vi "Rotate Pattern.vi"(9 "Target":i32, 10 "Current":i32, 11 "Pattern In":bool[][](array[boolean])) -> (2 "Rotation CCW":i32, 3 "Pattern Out":bool[][](array[boolean]))   [LabVIEW 2020]
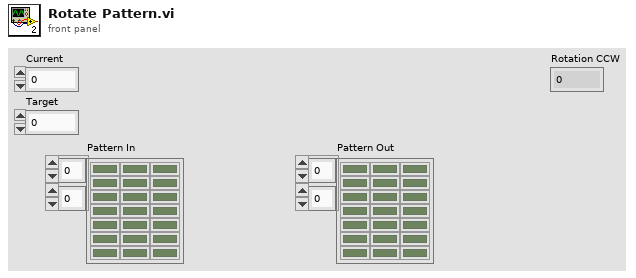
[diagram p1: front panel]
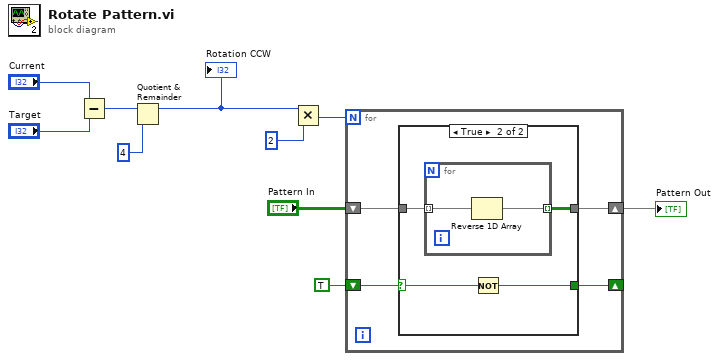
[diagram p0: block diagram]
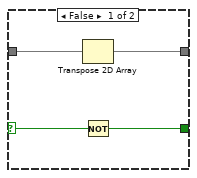
[diagram p2: hidden frame]
diagram:
  n1 = Subtract(x="Current", y="Target") -> (x-y=w8:i32)
  n2 = Quotient & Remainder(x=w8, y=4) -> (x-y*floor(x/y)=w6:i32)  [unwired: 1 out]
  "Rotation CCW" <- w6
  n3 = Multiply(x=w6, y=2) -> (x*y=w5:i32)
  n4 = for {
    N: w5 -> [_]
    shift-right: [w12] -> w1
    shift-left: "Pattern In" -> [w11]
    shift-right: [w13] -> _
    shift-left: TRUE -> [w14]
    n5 = case shown="True" w14 {
      selector: w14 -> [w18 w22]
      tunnel: [w17 w21] -> w13
      tunnel: [w15 w19] -> w12
      tunnel: w11 -> [w16 w20]
      frame False {
        n6 = Transpose 2D Array(2D array=w16) -> (transposed array=w15:bool[][])
        n7 = Not(x=w18) -> (.not. x?=w17:bool)
      }
      frame True {
        n8 = for {
          tunnel: w20 -> [w24] mode=indexing
          tunnel: [w23] -> w19 mode=indexing
          n9 = Reverse 1D Array(array=w24) -> (reversed array=w23:bool[])
        }
        n10 = Not(x=w22) -> (.not. x?=w21:bool)
      }
    }
  }
  "Pattern Out" <- w1
